vi "Functional Global Variable.vi"(8 "error in (no error)":errorcluster, 9 "Action":T1, 10 "Var name":string, 11 "Initialize to":string) -> (0 "error out":errorcluster, 3 "Result":string)   [LabVIEW 2013]
doc: "This VI is a Functional Global Variable that will take an initial value from the user, store it in the shift register, increment it then display the result in an indicator"
uses:
  Action Items.ctl
panel:
  in  "Var Data":string[](array[string])
  in  "Var Names":string[](array[string])
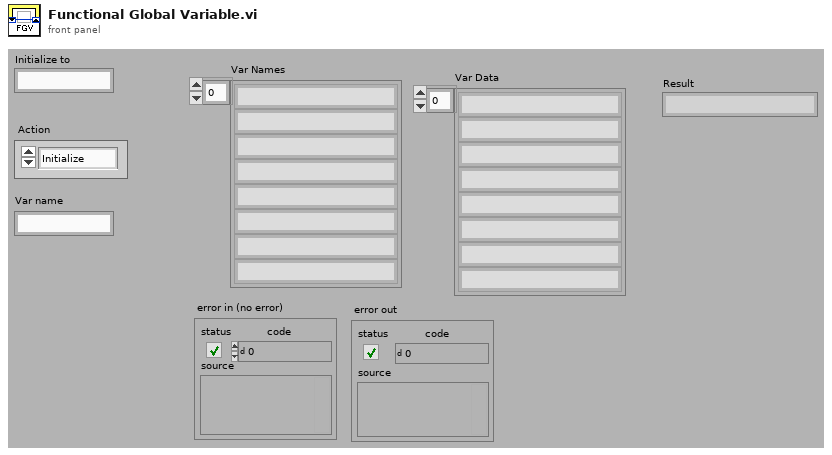
[diagram p1: front panel]
types:
  T1 = typedef "Action Items.ctl" = enum16{"Initialize", "Get", "Increment", "Set", "Clear table"}
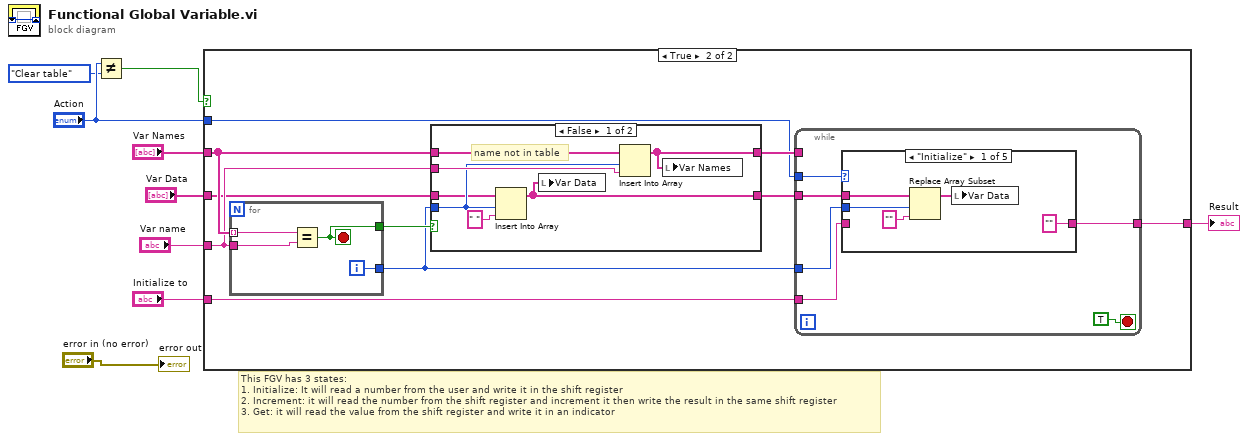
[diagram p0: block diagram]
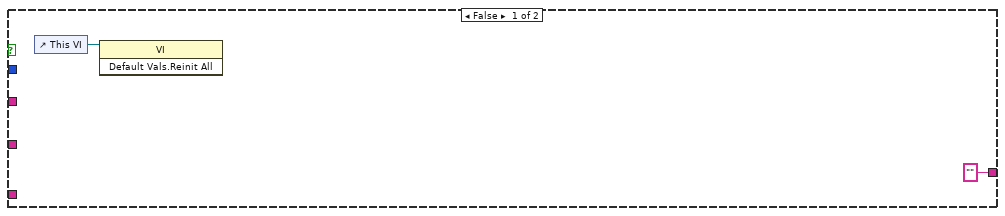
[diagram p2: hidden frame]
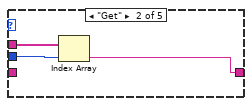
[diagram p4: hidden frame]
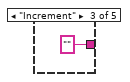
[diagram p5: hidden frame]
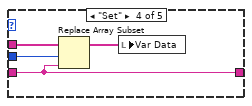
[diagram p6: hidden frame]
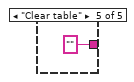
[diagram p7: hidden frame]
diagram:
  # "This FGV has 3 states:\n1. Initialize: It will read a number from the user and write it in the shift register\n2. Increment: it will read the number from the shift register and increment it then write the result in the same shift register\n3. Get: it will read the value from the shift register and write it in an indicator"
  n1 = Not Equal?(x="Action", y=Action_Items."Clear table") -> (x != y?=w2:bool)
  n2 = case shown="True" w2 {
    tunnel: "Var Names" -> [_ w20]
    tunnel: "Var name" -> [_ w19]
    tunnel: "Initialize to" -> [_ w17]
    tunnel: ["" ("Initialize to") w16] -> w6
    tunnel: "Var Data" -> [_ w14]
    tunnel: "Action" -> [_ w12]
    frame False {
      n3 = control-ref of="This VI"() -> (w11:refnum<vi>)
      n4 = invoke class="VI" method="Default Vals.Reinit All"(reference=w11) -> ()  [unwired: 2 in, 3 out]
    }
    frame True {
      n5 = for {
        tunnel: w20 -> [w34] mode=indexing
        tunnel: w19 -> [w33]
        tunnel: [w32] -> w18
        tunnel: [w31] -> w21
        i -> [w32]
        stop <- w31 stop-if-true
        n6 = Equal?(x=w34, y=w33) -> (x = y?=w31:bool)
      }
      n7 = case shown="False" w21 {
        tunnel: w20 -> [w28 w30]
        tunnel: w18 -> [w25 _]
        tunnel: w19 -> [w27 _]
        tunnel: [w26 w30] -> w15
        tunnel: w14 -> [w23 w29]
        tunnel: [w22 w29] -> w13
        frame False {
          # "name not in table"
          n8 = Insert Into Array(array=w23, index=w25, new element=" " ("new element/subarray")) -> (w22:string[])
          n9 = local write "Var Data"(w22) -> ()
          n10 = Insert Into Array(array=w28, index=w25, new element=w27) -> (w26:string[])
          n11 = local write "Var Names"(w26) -> ()
        }
        frame True {
        }
      }
      n12 = while {
        tunnel: w17 -> [w39]
        tunnel: w13 -> [w38]
        tunnel: w18 -> [w37]
        tunnel: [w36] -> w16
        tunnel: w15 -> [_]
        tunnel: w12 -> [w35]
        stop <- TRUE ("stop") stop-if-true
        n13 = case shown="\"Initialize\"" w35 {
          tunnel: ["" ("Initialize to") w46 "" ("Initialize to") w51 "" ("Initialize to")] -> w36
          tunnel: w39 -> [_ _ _ w51 _]
          tunnel: w38 -> [w44 w48 _ w53 _]
          tunnel: w37 -> [w43 w47 _ w52 _]
          frame "Initialize" {
            n14 = Replace Array Subset(array=w44, new element="" ("new element/subarray"), index=w43) -> (w45:string[])
            n15 = local write "Var Data"(w45) -> ()
          }
          frame "Get" {
            n16 = Index Array(array=w48, index=w47) -> (element=w46:string)
          }
          frame "Increment" {
          }
          frame "Set" {
            n17 = Replace Array Subset(array=w53, new element=w51, index=w52) -> (w50:string[])
            n18 = local write "Var Data"(w50) -> ()
          }
          frame "Clear table" {
          }
        }
      }
    }
  }
  "Result" <- w6
  "error out" <- "error in (no error)"
